vi "Conveyer Belt Control.vi"(8 "Frisbee States":T1, 11 "conveyer belt control":dbl) -> (0 "middle filled":bool, 1 "flipper filled":bool, 2 "conveyer belt":dbl)   [LabVIEW 2012]
uses:
  BotStatus.vi
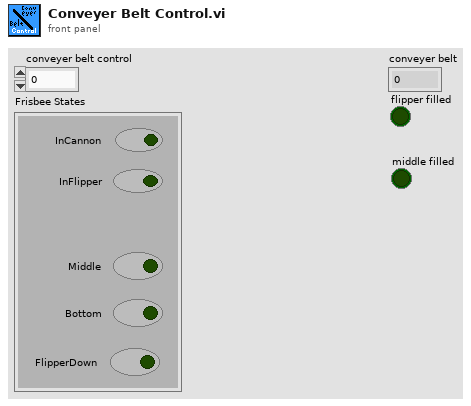
[diagram p1: front panel]
types:
  T1 = cluster{"Middle":bool, "InCannon":bool, "InFlipper":bool, "Bottom":bool, "FlipperDown":bool}
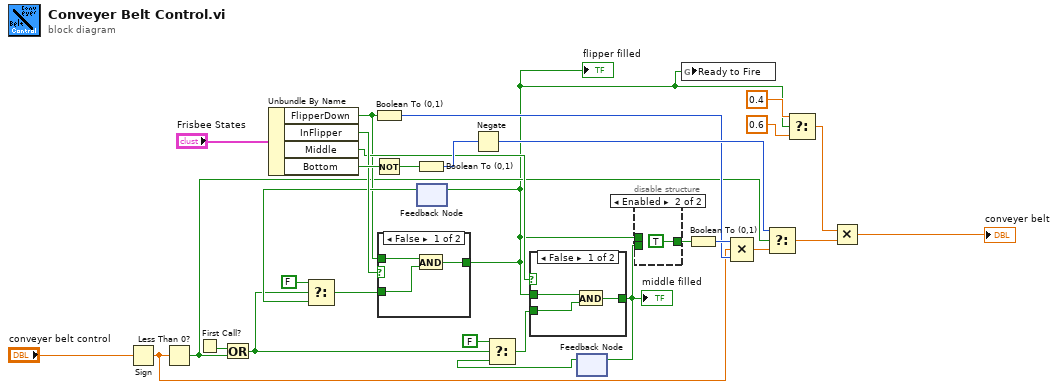
[diagram p0: block diagram]
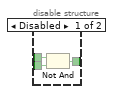
[diagram p2: hidden frame]
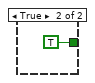
[diagram p3: hidden frame]
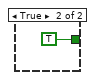
[diagram p4: hidden frame]
diagram:
  n1 = Sign(1:"conveyer belt control") -> (0:w8:dbl)
  n2 = Less Than 0?(x=w8) -> (x < 0?=w7:bool)
  n3 = First Call?() -> (First Call?: T/F=w17:bool)
  n4 = Or(x=w17, y=w7) -> (x .or. y?=w6:bool)
  n5 = Unbundle By Name("Frisbee States") -> ("FlipperDown"=w10:bool, "InFlipper"=w23:bool, "Middle"=w16:bool, "Bottom"=w28:bool)
  n6 = Boolean To (0,1)(Boolean=w10) -> (0, 1=w11:i16)
  n7 = Not(x=w28) -> (.not. x?=w29:bool)
  n8 = Boolean To (0,1)(Boolean=w29) -> (0, 1=w27:i16)
  n9 = feedback #1() -> (w22:bool)  [unwired: 1 in]
  n10 = Select(t=FALSE, s=w6, f=w22) -> (s? t:f=w20:bool)
  n11 = case shown="False" w23 {
    tunnel: [w31 TRUE] -> w1
    tunnel: w20 -> [w33 _]
    tunnel: w10 -> [w32 _]
    frame False {
      n12 = And(x=w32, y=w33) -> (x .and. y?=w31:bool)
    }
    frame True {
    }
  }
  "flipper filled" <- w1
  n13 = feedback-in #1(w1) -> ()
  n14 = Negate(x=w27) -> (-x=w24:i16)
  n15 = feedback #2() -> (w15:bool)  [unwired: 1 in]
  n16 = Select(t=FALSE, s=w6, f=w15) -> (s? t:f=w14:bool)
  n17 = case shown="False" w16 {
    tunnel: w1 -> [w35 _]
    tunnel: w14 -> [w37 _]
    tunnel: [w36 TRUE ("t")] -> w12
    frame False {
      n18 = And(x=w35, y=w37) -> (x .and. y?=w36:bool)
    }
    frame True {
    }
  }
  "middle filled" <- w12
  n19 = feedback-in #2(w12) -> ()
  n20 = disable-structure shown="Enabled" {
    disable-tunnel: [w41 TRUE] -> w13
    disable-tunnel: w12 -> [w40 _]
    disable-tunnel: w1 -> [w39 _]
    frame Disabled {
      n21 = Not And(1:w40, 2:w39) -> (0:w41:bool)
    }
    frame Enabled {
    }
  }
  n22 = global write "BotStatus.vi" "Ready to Fire"(w1) -> ()
  n23 = Boolean To (0,1)(Boolean=w13) -> (0, 1=w30:i16)
  n24 = Compound Arithmetic op=MULTIPLY(w30, w8, w11) -> (w26:dbl)
  n25 = Select(t=w24, s=w7, f=w26) -> (s? t:f=w25:dbl)
  n26 = Select(t=0.4, s=w1, f=0.6) -> (s? t:f=w3:dbl)
  n27 = Multiply(x=w3, y=w25) -> (x*y=→"conveyer belt":dbl)
